vi "TCP Server.vi"() -> ()   [LabVIEW 2011]
uses:
  <vilib>/STM32_DriverVI_Interface_F4/Ethernet/IP Type_F4.ctl
panel:
  out "数值":i32
  out "返回字符串":string
  out "Read_Valid?":bool
  in  "发送字符串":string
  out "Send_Valid?":bool
  out "Init_Success?":bool
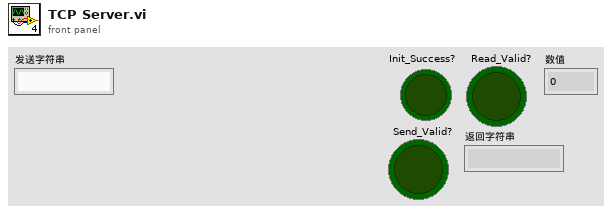
[diagram p1: front panel]
types:
  T1 = typedef "IP Type_F4.ctl" = enum8{"Host IP Address", "Gateway Address", "Subnet Mask Address"}
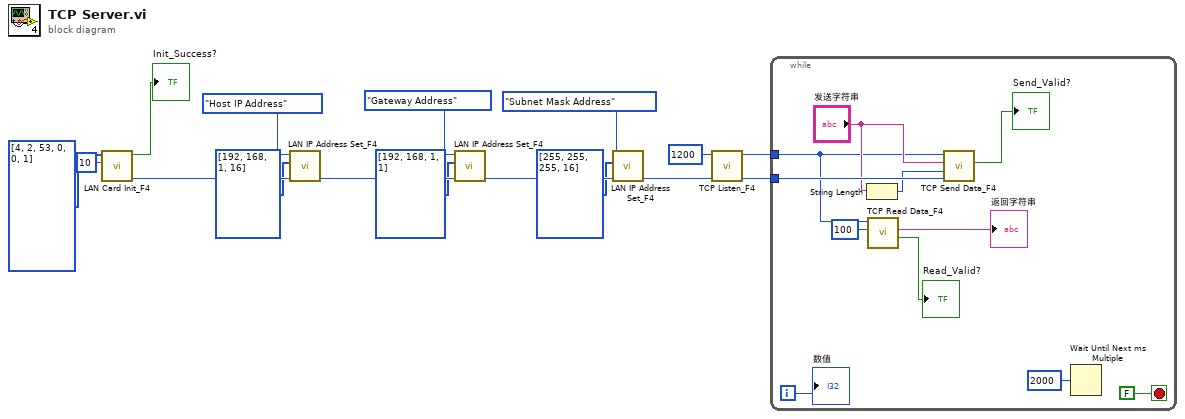
[diagram p0: block diagram]
diagram:
  n1 = call <vilib>:"LAN Card Init_F4.vi"("Scan_Engine（ms）"=u16 10, "MAC_Address（Hex）"=u8[] [4, 2, 53, 0, 0, 1]) -> ("err_out"=w13:u8, "Init_Success?"=→"Init_Success?":bool)  [unwired: 8 in]
  n2 = call <vilib>:"LAN IP Address Set_F4.vi"("err_in"=w13, "IP_Address（Decimal）"=u8[] [192, 168, 1, 16], "IP Address Type"=IP_Type_F4."Host IP Address") -> ("err_out"=w10:u8)  [unwired: 8 in]
  n3 = call <vilib>:"LAN IP Address Set_F4.vi"("err_in"=w10, "IP_Address（Decimal）"=u8[] [192, 168, 1, 1], "IP Address Type"=IP_Type_F4."Gateway Address") -> ("err_out"=w7:u8)  [unwired: 8 in]
  n4 = call <vilib>:"LAN IP Address Set_F4.vi"("err_in"=w7, "IP_Address（Decimal）"=u8[] [255, 255, 255, 16], "IP Address Type"=IP_Type_F4."Subnet Mask Address") -> ("err_out"=w4:u8)  [unwired: 8 in]
  n5 = call <vilib>:"TCP Listen_F4.vi"("err_in"=w4, "Local Port"=u16 1200) -> ("err_out"=w2:u8, "Connect_ID"=w1:u8)  [unwired: 8 in]
  n6 = while {
    tunnel: w2 -> [w27]
    tunnel: w1 -> [w23]
    i -> [w17]
    stop <- FALSE stop-if-true
    n7 = String Length(string="发送字符串") -> (length=w25:i32)
    n8 = call <vilib>:"TCP Read Data_F4.vi"("Read_Number（0~1024）"=u16 100, "Connect_ID"=w23) -> ("Read_Valid?"=→"Read_Valid?":bool, "返回字符串"=→"返回字符串":string)  [unwired: 4 in, 4 out]
    n9 = call <vilib>:"TCP Send Data_F4.vi"("err_in"=w27, "Send_Number（0~4096）"=w25, "发送字符串"="发送字符串", "Connect_ID"=w23) -> ("Send_Valid?"=→"Send_Valid?":bool)  [unwired: 5 in, 2 out]
    n10 = Wait Until Next ms Multiple(millisecond multiple=u32 2000 ("毫秒倍数")) -> ()  [unwired: 1 out]
    "数值" <- w17
  }
